vi "DSF.Engine.BuilderManager.Get Builder.vi"(10 "ID":i32, 11 "Builder Manager in":refnum<class "DSF.Engine.BuilderManager.lvclass">) -> (2 "Builder":refnum<class "DSF.Engine.Builder.lvclass">, 3 "Builder Manager out":refnum<class "DSF.Engine.BuilderManager.lvclass">)   [LabVIEW 2017, in "DSF.Engine.lvlib" / "DSF.Engine.BuilderManager.lvclass"]
uses:
  DSF.Engine.BuilderManager.lvclass
  Builder/DSF.Engine.Builder.lvclass
  DSF.Engine.BuilderManager.lvclass/DSF.Engine.BuilderManager.ctl
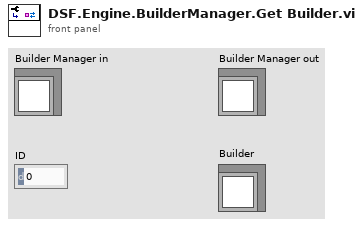
[diagram p1: front panel]
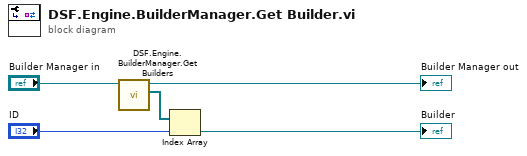
[diagram p0: block diagram]
diagram:
  n1 = call "DSF.Engine.BuilderManager.Get Builders.vi"("Builder Manager in"="Builder Manager in") -> ("Builders"=w3:refnum<class "DSF.Engine.Builder.lvclass">[], "Builder Manager out"=→"Builder Manager out":refnum<class "DSF.Engine.BuilderManager.lvclass">)  [unwired: 9 in]
  n2 = Index Array(array=w3, index="ID") -> (element=→"Builder":refnum<class "DSF.Engine.Builder.lvclass">)
